vi "WaveFormToString.vi"(7 "channelName":string, 11 "Waveform":waveform(dbl)) -> (3 "string":string)   [LabVIEW 2013]
panel:
  out "double precision float":dbl
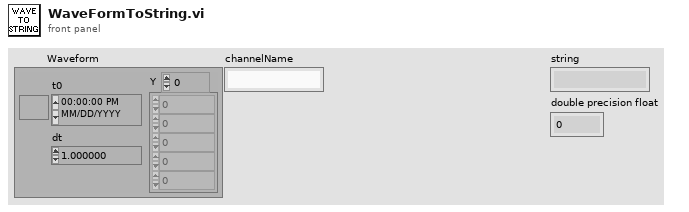
[diagram p1: front panel]
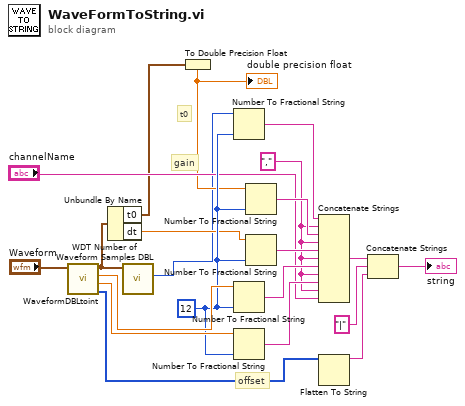
[diagram p0: block diagram]
diagram:
  w14 = i16 12 ("precision (6)")
  w4 = "," ("string")
  # "gain"
  # "offset"
  # "t0"
  n1 = call "WaveformDBLtoint.vi"("Waveform"="Waveform") -> ("32bit integer"=w19:i16[], "scale"=w21:dbl, "offset"=w20:dbl, "waveform out"=w7:waveform(dbl))  [unwired: 7 in]
  n2 = Unbundle By Name(w7) -> ("t0"=w5:timestamp, "dt"=w6:dbl)
  n3 = call "WDT Number of Waveform Samples DBL.vi"("waveform in"=w7) -> ("number of samples"=w1:i32)  [unwired: 8 in, 2 out]
  n4 = To Double Precision Float(number=w5) -> (double precision float=w2:dbl)
  "double precision float" <- w2
  n5 = Number To Fractional String(number=w1, precision (6)=w14) -> (F-format string=w3:string)  [unwired: 2 in]
  n6 = Number To Fractional String(number=w20, precision (6)=w14) -> (F-format string=w18:string)  [unwired: 2 in]
  n7 = Number To Fractional String(number=w21, precision (6)=w14) -> (F-format string=w13:string)  [unwired: 2 in]
  n8 = Number To Fractional String(number=w2, precision (6)=w14) -> (F-format string=w11:string)  [unwired: 2 in]
  n9 = Number To Fractional String(number=w6, precision (6)=w14) -> (F-format string=w12:string)  [unwired: 2 in]
  n10 = Concatenate Strings(w3, w4, w11, w4, w12, w4, w18, w4, w13, w4, "channelName") -> (w15:string)
  n11 = Flatten To String(anything=w19) -> (data string=w17:string)  [unwired: 3 in, 2 out]
  n12 = Concatenate Strings(w15, "|" ("string"), w17) -> (→"string":string)
